vi "Write HttpContent out.vi"(8 "error in (no error)":errorcluster, 10 "LabVIEWHTTPClient_NET.lvlib:HttpContent.lvclass":refnum<class "HttpContent.lvclass">, 11 "HttpDownloadTask in":refnum<class "HttpDownloadTask.lvclass">) -> (0 "error out":errorcluster, 3 "HttpDownloadTask out":refnum<class "HttpDownloadTask.lvclass">)   [LabVIEW 2018, in "HttpClient_NET.lvlib" / "HttpDownloadTask.lvclass"]
doc: "<b> </b> <b> </b>\nHttpClient_NET\nJustin Young - Viviota\nCopyright (c) 2021\nLicense: BSD"
uses:
  HttpDownloadTask.lvclass
  HttpContent/HttpContent.lvclass
  HttpDownloadTask.lvclass/HttpDownloadTask.ctl
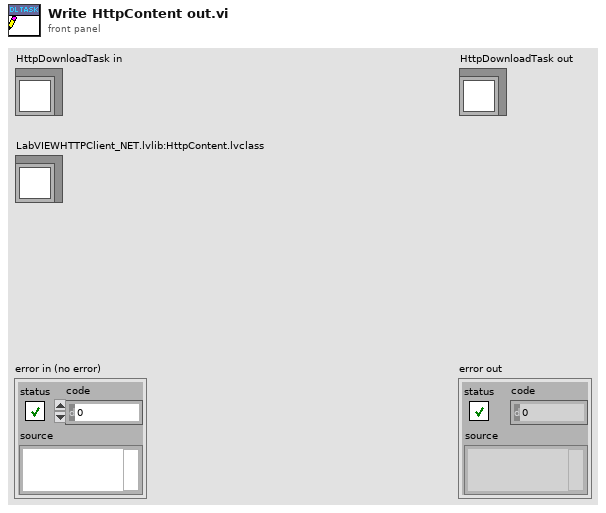
[diagram p1: front panel]
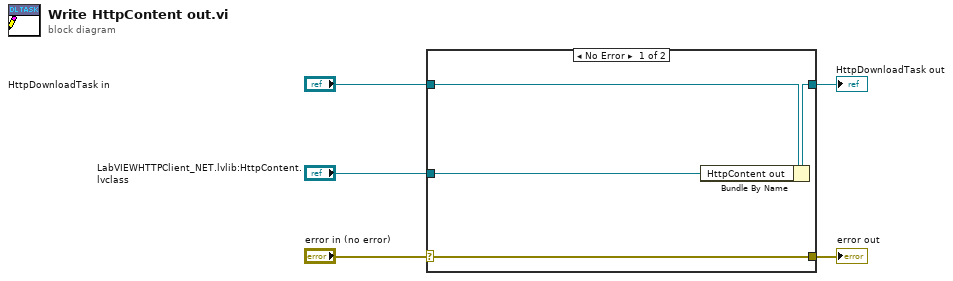
[diagram p0: block diagram]
diagram:
  n1 = case shown="No Error" "error in (no error)" {
    selector: "error in (no error)" -> [w9 w10]
    tunnel: [w9 w10] -> w4
    tunnel: [w7 w11] -> w2
    tunnel: "HttpDownloadTask in" -> [w8 w11]
    tunnel: "LabVIEWHTTPClient_NET.lvlib:HttpContent.lvclass" -> [w6 _]
    frame No Error {
      n2 = Bundle By Name(cluster=w8, "HttpContent out"=w6) -> (w7:refnum<class "HttpDownloadTask.lvclass">)
    }
    frame Error {
    }
  }
  "error out" <- w4
  "HttpDownloadTask out" <- w2
